vi "Continuous Decimating.vi"() -> ()   [LabVIEW 2023]
doc: "This example demonstrates how to use the Decimate (continuous) VI to process a large data sequence consisting of smaller blocks."
uses:
  <vilib>/Analysis/2dsp.llb/Decimate (continuous, DBL).vi
  <vilib>/Analysis/NI_AALBase.lvlib
  <vilib>/Analysis/NI_AALPro.lvlib
panel:
  out "Waveform Chart":waveform(dbl)[](graph)
  in  "Stop":bool
  in  "Decimating factor":i32(slide)=8 scale=1.0..10.0
  # "Overview: This example demonstrates how to use the Decimate (continuous) VI to process a large data sequence consisting of smaller blocks of data.\nRequirements: LabVIEW Full Development System\nInstructions:\n1. Run the VI.\n2. Change the Decimating factor and view the resulting decimated signal in the chart.\n3. Click Stop to stop the VI."
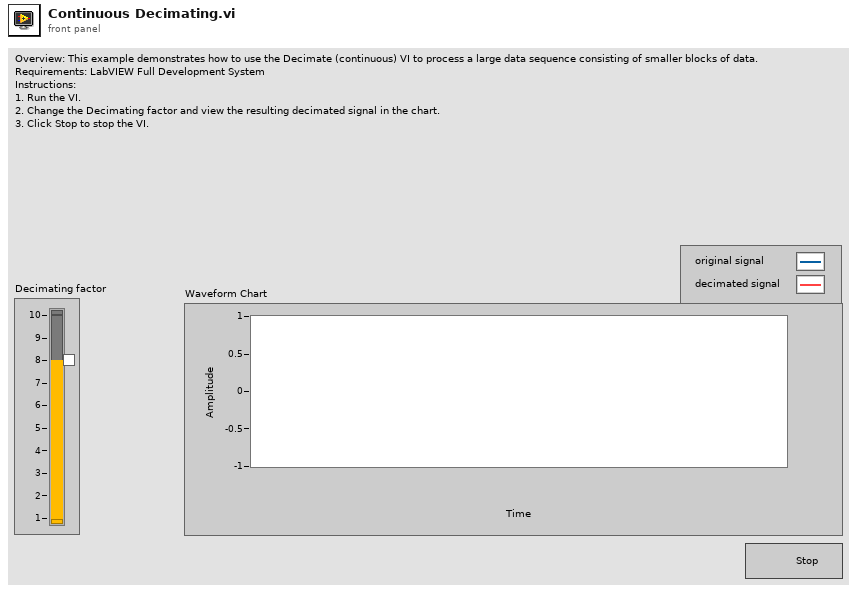
[diagram p1: front panel]
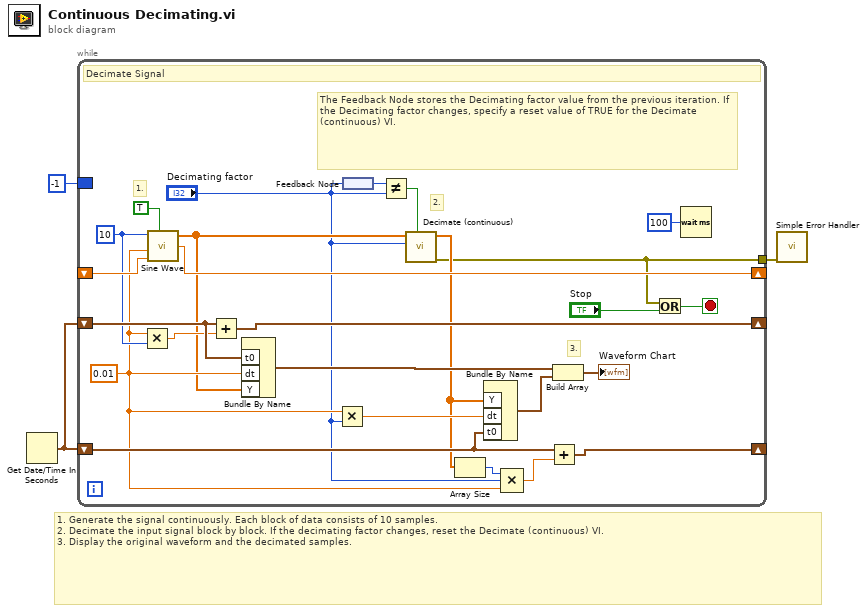
[diagram p0: block diagram]
diagram:
  # "1. Generate the signal continuously. Each block of data consists of 10 samples.\n2. Decimate the input signal block by block. If the decimating factor changes, reset the Decimate (continuous) VI.\n3. Display the original waveform and the decimated samples."
  n1 = Get Date/Time In Seconds() -> (seconds since 1Jan1904=w3:timestamp)
  n2 = while {
    shift-right: [w25] -> _
    shift-left: w3 -> [w28]
    shift-right: [w24] -> _
    shift-left: w3 -> [w23]
    shift-right: [w26] -> _
    shift-left: _ -> [w27]
    tunnel: [w9] -> w2
    border: -1 -> [_]
    stop <- w10 stop-if-true
    w14 = 0.01 ("frequency")
    w22 = 10 ("samples")
    # "The Feedback Node stores the Decimating factor value from the previous iteration. If the Decimating factor changes, specify a reset value of TRUE for the Decimate (continuous) VI."
    # "3."
    # "2."
    # "1."
    # "Decimate Signal"
    n3 = Multiply(x=w14, y=w22) -> (x*y=w21:dbl)
    n4 = call <vilib>:"Sine Wave.vi"("samples"=w22, "frequency"=w14, "phase in"=w27, "reset phase"=TRUE) -> ("sine wave"=w12:dbl[], "phase out"=w26:dbl)  [unwired: 1 in, 1 out]
    n5 = Add(x=w28, y=w21) -> (x+y=w25:timestamp)
    n6 = Bundle By Name("t0"=w28, "dt"=w14, "Y"=w12) -> (w20:waveform(dbl))  [unwired: 1 in]
    n7 = Multiply(x=w14, y="Decimating factor") -> (x*y=w15:dbl)
    n8 = feedback-in #1("Decimating factor") -> ()
    n9 = feedback #1() -> (w6:i32)
    n10 = Not Equal?(x=w6, y="Decimating factor") -> (x != y?=w4:bool)
    n11 = call-poly <vilib>:"Decimate (continuous).vi"("reset"=w4, "decimating factor"="Decimating factor", "X"=w12) -> ("error out"=w9:errorcluster, "Decimated Array"=w13:dbl[])  [unwired: 7 in]
    n12 = Array Size(array=w13) -> (size(s)=w18:i32)
    n13 = Bundle By Name("Y"=w13, "dt"=w15, "t0"=w23) -> (w19:waveform(dbl))  [unwired: 1 in]
    n14 = Compound Arithmetic op=MULTIPLY(w18, "Decimating factor", w14) -> (w17:dbl)
    n15 = Add(x=w23, y=w17) -> (x+y=w24:timestamp)
    n16 = Build Array(w20, w19) -> (→"Waveform Chart":waveform(dbl)[])
    n17 = Or(x=w9, y="Stop") -> (x .or. y?=w10:bool)
    n18 = Wait (ms)(milliseconds to wait=u32 100) -> ()  [unwired: 1 out]
  }
  n19 = call <vilib>:"Simple Error Handler.vi"("error in (no error)"=w2) -> ()  [unwired: 4 in, 5 out]
